vi "Void_request.vi"(8 "error in (no error)":errorcluster, 10 "SQL request":string, 11 "DB_SQLite in":refnum<class "DB_SQLite.lvclass">) -> (0 "error out":errorcluster, 3 "DB_SQLite out":refnum<class "DB_SQLite.lvclass">)   [LabVIEW 2020, in "DB_SQLite.lvclass"]
uses:
  DB_SQLite.lvclass
  C:/dev/TRANCON/Classes/DB/DB.lvclass
  DB.lvclass/DB.ctl
  <vilib>/drjdpowell/SQLite Library/SQL Connection/Execute SQL (No results).vi
  <vilib>/drjdpowell/SQLite Library/SQLite.lvlib
  <vilib>/drjdpowell/SQLite Library/SQL Connection/Connection.lvclass
  DB.lvclass
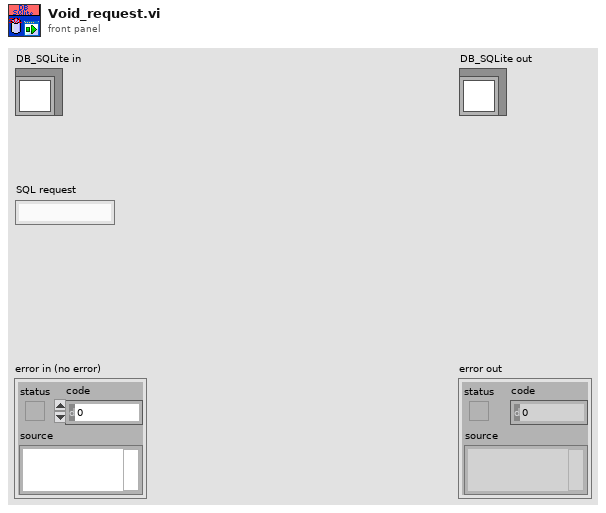
[diagram p1: front panel]
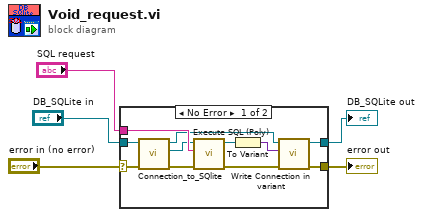
[diagram p0: block diagram]
diagram:
  n1 = case shown="No Error" "error in (no error)" {
    selector: "error in (no error)" -> [w10 w18]
    tunnel: [w13 w18] -> w4
    tunnel: [w11 w17] -> w3
    tunnel: "DB_SQLite in" -> [w9 w17]
    tunnel: "SQL request" -> [w16 _]
    frame No Error {
      n2 = call "Connection_to_SQlite.vi"("error in (no error)"=w10, "DB_SQLite in"=w9) -> ("error out"=w6:errorcluster, "SQlite connection"=w7:refnum<class "Connection.lvclass">, "DB_SQLite out"=w8:refnum<class "DB_SQLite.lvclass">)  [unwired: 7 in]
      n3 = call-poly <vilib>:"Execute SQL (Poly).vi"("error in (no error)"=w6, "SQL"=w16, "SQLite Connection in"=w7) -> ("error out"=w14:errorcluster, "SQLite Connection"=w15:refnum<class "Connection.lvclass">)  [unwired: 7 in]
      n4 = To Variant(anything=w15) -> (Variant=w12:variant)
      n5 = call "Write Connection in variant.vi"("error in (no error)"=w14, "Connection in variant"=w12, "DB in"=w8) -> ("error out"=w13:errorcluster, "DB out"=w11:refnum<class "DB_SQLite.lvclass">)  [unwired: 7 in]
    }
    frame Error {
    }
  }
  "error out" <- w4
  "DB_SQLite out" <- w3
